vi "Standard table polymorphic.vi"   [LabVIEW 2019]
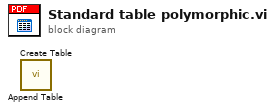
[diagram p0: block diagram]
diagram:
  n1 = call <userlib>:"Append Table.vi"() -> ()  [unwired: 14 in, 2 out]
  n2 = call <userlib>:"Create Table.vi"() -> ()  [unwired: 13 in, 3 out]
